vi "Image Display_Copy Image to Clipboard.vi"(8 "Error In":errorcluster, 9 "Image to Clipboard Options":T1={"Include Overlay (T)"=TRUE, "Image Only (T)"=TRUE}, 11 "Display Image Control Refnum":T2) -> (0 "Error Out":errorcluster)   [LabVIEW 2021]
uses:
  Image Control Refnum.ctl
  Image Display to Clipboard Options.ctl
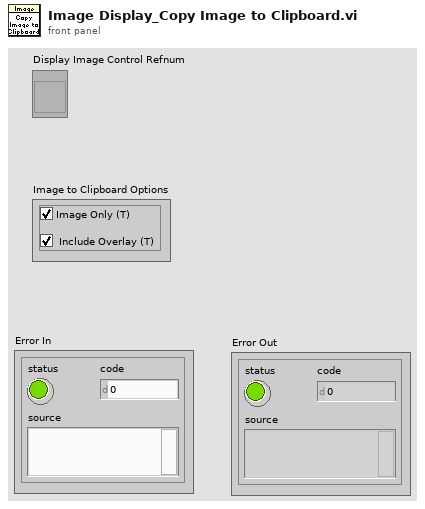
[diagram p1: front panel]
types:
  T1 = typedef "Image Display to Clipboard Options.ctl" = cluster{"Include Overlay (T)":bool, "Image Only (T)":bool}
  T2 = typedef "Image Control Refnum.ctl" = refnum<vi>
  T3 = typedef "imagedata.ctl" = cluster{"image type":i32, "image depth":i32, "image":u8[], "mask":u8[], "colors":u32[], "Rectangle":cluster{"left":i16, "top":i16, "right":i16, "bottom":i16}}
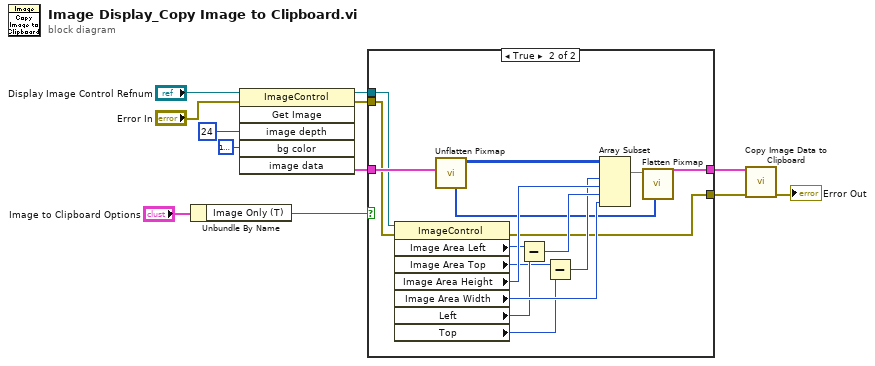
[diagram p0: block diagram]
diagram:
  n1 = Unbundle By Name("Image to Clipboard Options") -> ("Image Only (T)"=w6:bool)
  n2 = invoke class="ImageControl" method="Get Image"(reference="Display Image Control Refnum", error in="Error In", "image depth"=24 ("Image Depth"), "bg color"=u32 16777226 ("Background Color")) -> (reference out=w1:T2, error out=w5:errorcluster, "image data"=w3:T3)  [unwired: 2 in, 3 out]
  n3 = case shown="True" w6 {
    tunnel: w5 -> [w14 w17]
    tunnel: [w14 w16] -> w4
    tunnel: w3 -> [w13 w19]
    tunnel: [w13 w15] -> w2
    tunnel: w1 -> [_ w18]
    frame False {
    }
    frame True {
      n4 = property class="ImageControl"(reference=w18, error in=w17) -> (error out=w16:errorcluster, "Image Area Left"=w21:i32, "Image Area Top"=w22:i32, "Image Area Height"=w29:u32, "Image Area Width"=w30:u32, "Left"=w25:i32, "Top"=w26:i32)  [unwired: 1 out]
      n5 = call <vilib>:"Unflatten Pixmap.vi"("image data"=w19) -> ("24-bit pixmap"=w20:u32[][], "colors"=w24:u32[])  [unwired: 4 in, 5 out]
      n6 = Subtract(x=w21, y=w25) -> (x-y=w28:i32)
      n7 = Subtract(x=w22, y=w26) -> (x-y=w27:i32)
      n8 = Array Subset(array=w20, index (row)=w27, length (row)=w29, index (col)=w28, length (col)=w30) -> (w23:u32[][])
      n9 = call <vilib>:"Flatten Pixmap.vi"("colors"=w24, "24-bit pixmap"=w23) -> ("image data"=w15:T3)  [unwired: 9 in]
    }
  }
  n10 = call "Copy Image Data to Clipboard.vi"("error in (no error)"=w4, "image data"=w2) -> ("error out"=→"Error Out":errorcluster)  [unwired: 9 in]
